vi "Handle Notification.vi"(8 "error in (no error)":errorcluster, 9 "Payload":string, 10 "Notification Type":string, 11 "Historical Table in":refnum<class "Historical Table.lvclass">) -> (0 "error out":errorcluster, 3 "Historical Table out":refnum<class "Historical Table.lvclass">)   [LabVIEW 2024, in "Historical Table.lvlib" / "Historical Table.lvclass"]
uses:
  Historical Table.lvclass
  Historical Table.lvclass/Historical Table.ctl
  Global Strings.vi
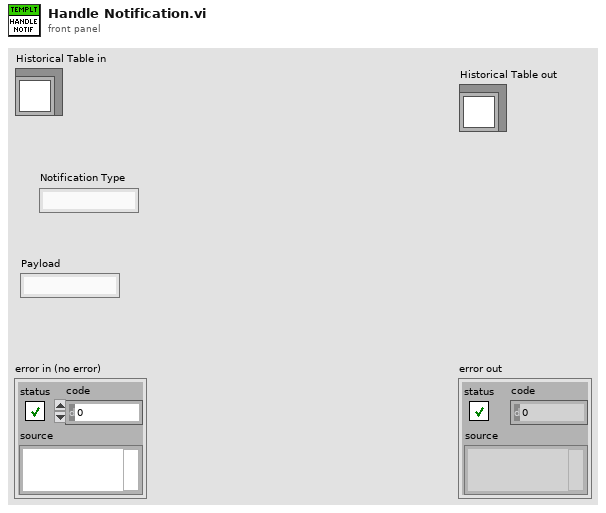
[diagram p1: front panel]
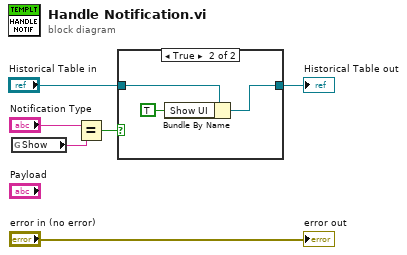
[diagram p0: block diagram]
diagram:
  n1 = global read "Global Strings.vi" "Show"() -> (w6:string)
  n2 = Equal?(x="Notification Type", y=w6) -> (x = y?=w5:bool)
  n3 = case shown="True" w5 {
    tunnel: "Historical Table in" -> [w7 w10]
    tunnel: [w7 w8] -> w1
    frame False {
    }
    frame True {
      n4 = Bundle By Name(cluster=w10, "Show UI"=TRUE) -> (w8:refnum<class "Historical Table.lvclass">)
    }
  }
  "Historical Table out" <- w1
  "error out" <- "error in (no error)"
